vi "240126_Change_XY_Position.vi"(0 "Relative move (mm)":dbl=1.0, 5 "Position in":dbl[](array[numeric])=[0.0, 0.0], 7 "-+ (FT)":bool, 9 "XY (0-1)":u8, 11 "error in (no error)":errorcluster) -> (4 "Position out":dbl[](array[numeric])=[1.0, 0.0], 15 "error out":errorcluster)   [LabVIEW 2023]
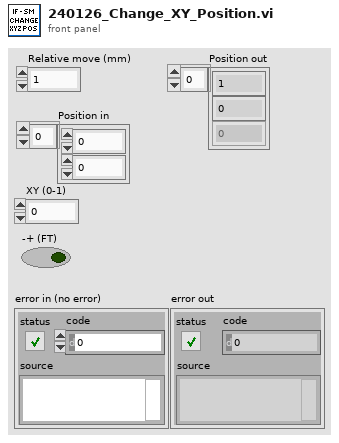
[diagram p1: front panel]
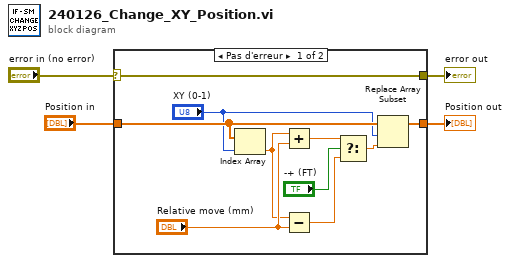
[diagram p0: block diagram]
diagram:
  n1 = case shown="Pas d'erreur" "error in (no error)" {
    selector: "error in (no error)" -> [w14 w16]
    tunnel: [w14 w16] -> w3
    tunnel: "Position in" -> [w13 w15]
    tunnel: [w12 w15] -> w1
    frame No Error {
      n2 = Index Array(array=w13, index="XY (0-1)") -> (element=w6:dbl)
      n3 = Add(x=w6, y="Relative move (mm)") -> (x+y=w5:dbl)
      n4 = Subtract(x=w6, y="Relative move (mm)") -> (x-y=w8:dbl)
      n5 = Select(t=w5, s="-+ (FT)", f=w8) -> (s? t:f=w10:dbl)
      n6 = Replace Array Subset(array=w13, new element=w10, index="XY (0-1)") -> (w12:dbl[])
    }
    frame Error {
    }
  }
  "Position out" <- w1
  "error out" <- w3
